vi "Class to Variant.vi"(8 "error in (no error)":errorcluster, 10 "Data in":variant, 11 "Serializable Node in":refnum<class "Serializable Node.lvclass">) -> (0 "error out":errorcluster, 1 "Serialized Object Name":string, 2 "Data Out":variant, 3 "Serializable Node out":refnum<class "Serializable Node.lvclass">)   [LabVIEW 2014, in "Serializable Node.lvclass"]
uses:
  Serializable Node.lvclass
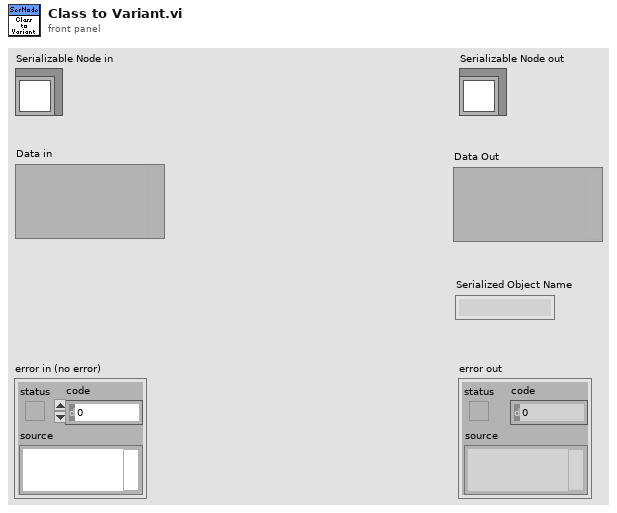
[diagram p1: front panel]
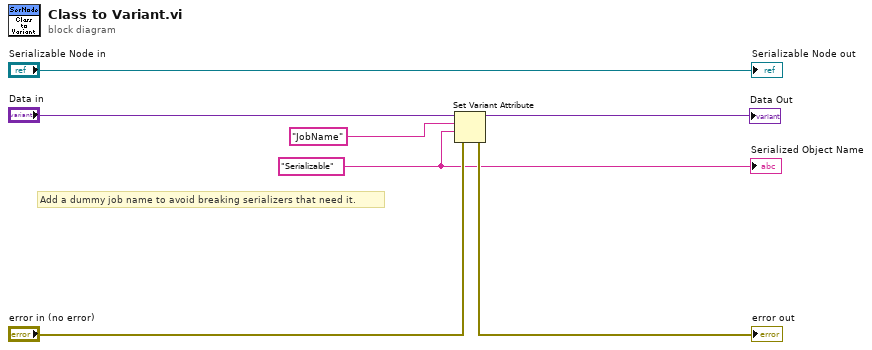
[diagram p0: block diagram]
diagram:
  w1 = "Serializable" ("name")
  # "Add a dummy job name to avoid breaking serializers that need it."
  n1 = Set Variant Attribute(Variant="Data in", name="JobName", value=w1, error in="error in (no error)") -> (Variant out=→"Data Out":variant, error out=→"error out":errorcluster)  [unwired: 1 out]
  "Serializable Node out" <- "Serializable Node in"
  "Serialized Object Name" <- w1
